vi "LOAD_CONFIG.vi"() -> (3 "출력 클러스터":T1)   [LabVIEW 2019]
uses:
  <vilib>/imath/engines/lvmath/Plug In/Control Design/BuiltInFunctions/tf/NIMS_CD_tf(num,den,Ts).vi
  <vilib>/imath/engines/lvmath2/RunTimeEngine/NodeEndStatement/NIMS_NodeEndStatement_Output.vi
  <vilib>/imath/engines/lvmath2/RunTimeEngine/ErrorHandling/NIMS_Finalize Error.vi
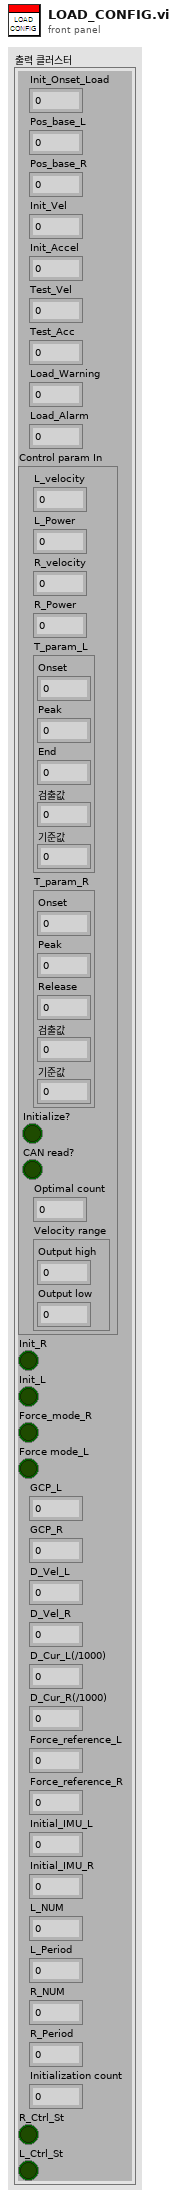
[diagram p1: front panel]
types:
  T1 = cluster{"Init_Onset_Load":sgl, "Pos_base_L":sgl, "Pos_base_R":sgl, "Init_Vel":i32, "Init_Accel":u32, "Test_Vel":i32, "Test_Acc":u32, "Load_Warning":sgl, "Load_Alarm":sgl, "Control param In":cluster{"L_velocity":u32, "L_Power":sgl, "R_velocity":u32, "R_Power":sgl, "T_param_L":cluster{"Onset":sgl, "Peak":sgl, "End":sgl, "검출값":sgl, "기준값":sgl}, "T_param_R":cluster{"Onset":sgl, "Peak":sgl, "Release":sgl, "검출값":sgl, "기준값":sgl}, "Initialize?":bool, "CAN read?":bool, "Optimal count":i32, "Velocity range":cluster{"Output high":dbl, "Output low":dbl}}, "Init_R":bool, "Init_L":bool, "Force_mode_R":bool, "Force mode_L":bool, "GCP_L":sgl, "GCP_R":sgl, "D_Vel_L":sgl, "D_Vel_R":sgl, "D_Cur_L(/1000)":sgl, "D_Cur_R(/1000)":sgl, "Force_reference_L":sgl, "Force_reference_R":sgl, "Initial_IMU_L":sgl, "Initial_IMU_R":sgl, "L_NUM":u32, "L_Period":i16, "R_NUM":u32, "R_Period":i16, "Initialization count":i32, "R_Ctrl_St":bool, "L_Ctrl_St":bool}
  T2 = cluster{"Init_Onset_Load":sgl, "Pos_base_L":sgl, "Pos_base_R":sgl, "Init_Vel":i32, "Init_Accel":u32, "Test_Vel":i32, "Test_Acc":u32, "Load_Warning":sgl, "Load_Alarm":sgl, "Control param In":cluster{"L_velocity":u32, "L_Power":sgl, "R_velocity":u32, "R_Power":sgl, "T_param_L":cluster{"Onset":sgl, "Peak":sgl, "End":sgl, "검출값":sgl, "기준값":sgl}, "T_param_R":cluster{"Onset":sgl, "Peak":sgl, "Release":sgl, "검출값":sgl, "기준값":sgl}, "Initialize?":bool, "CAN read?":bool, "Optimal count":i32, "Velocity range":cluster{"Output high":dbl, "Output low":dbl}}}
  T3 = cluster{"L_velocity":u32, "L_Power":sgl, "R_velocity":u32, "R_Power":sgl, "T_param_L":cluster{"Onset":sgl, "Peak":sgl, "End":sgl, "검출값":sgl, "기준값":sgl}, "T_param_R":cluster{"Onset":sgl, "Peak":sgl, "Release":sgl, "검출값":sgl, "기준값":sgl}, "Initialize?":bool, "CAN read?":bool, "Optimal count":i32, "Velocity range":cluster{"Output high":dbl, "Output low":dbl}}
  T4 = enum16{"open", "replace", "create", "open or create", "replace or create", "replace or create with confirmation"}
  T5 = cluster{"Onset":sgl, "Peak":sgl, "End":sgl, "검출값":sgl, "기준값":sgl}
  T6 = cluster{"Onset":sgl, "Peak":sgl, "Release":sgl, "검출값":sgl, "기준값":sgl}
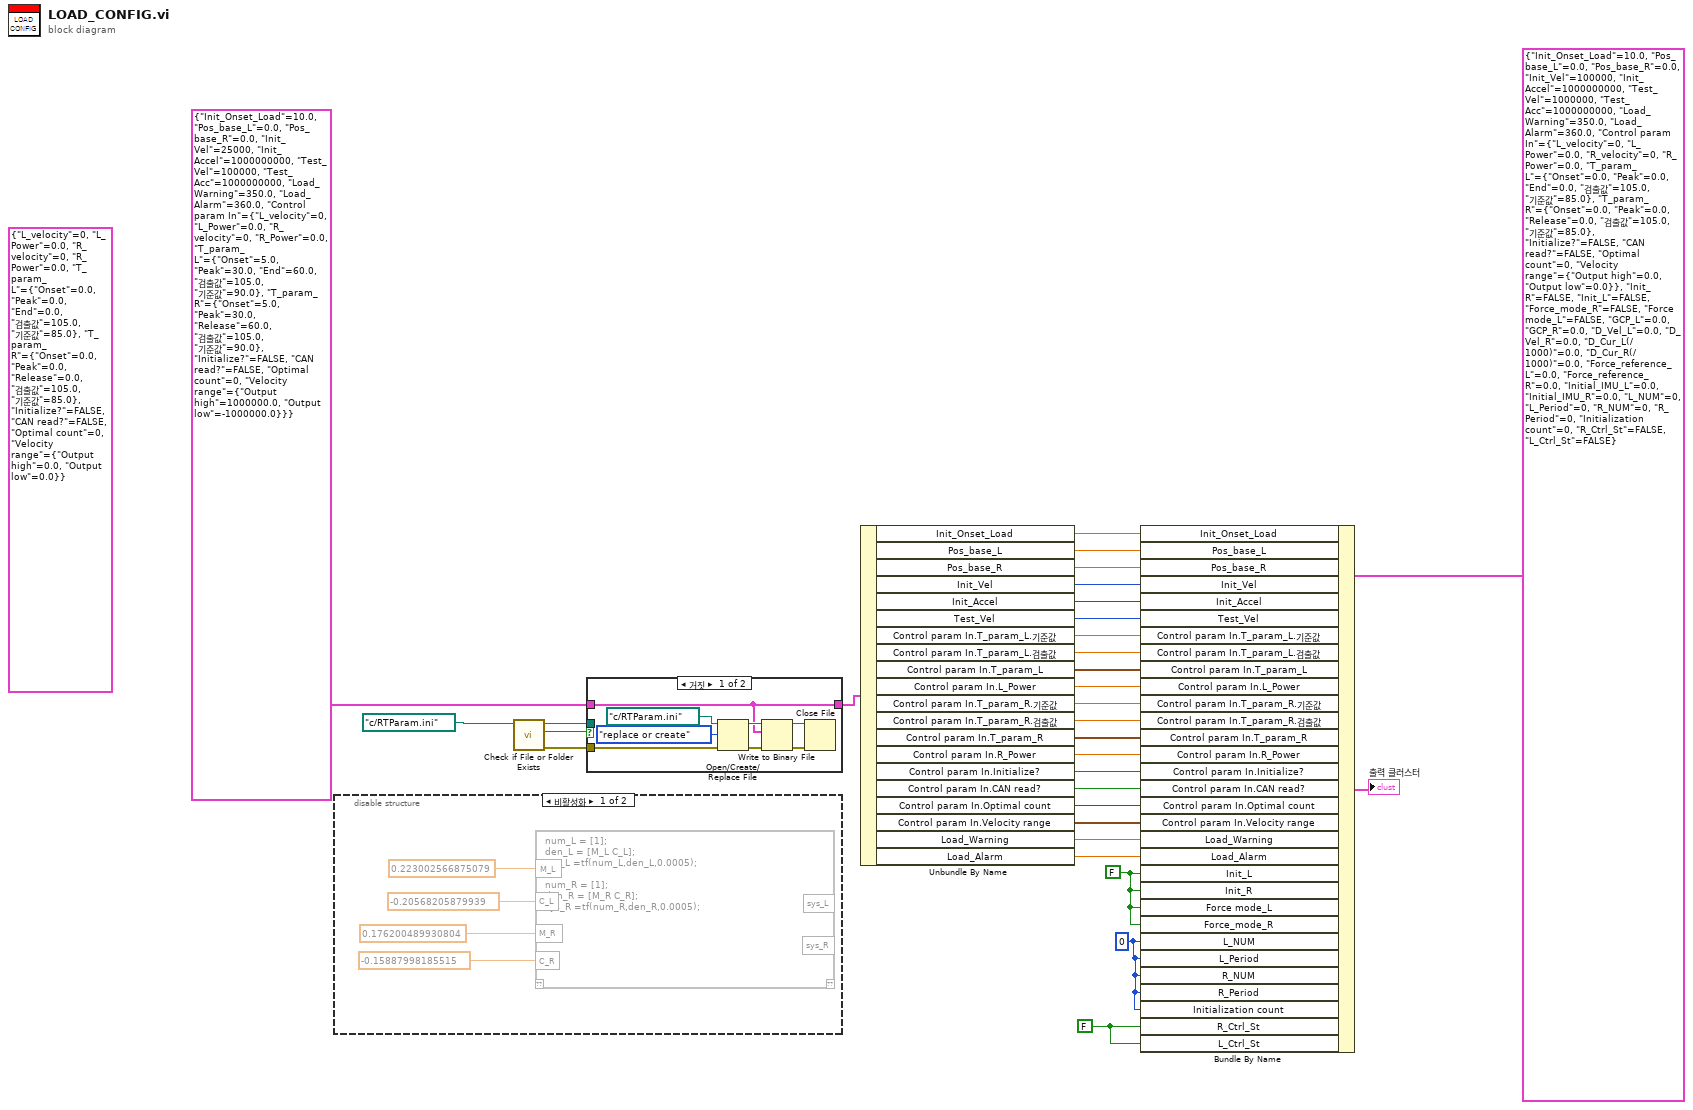
[diagram p0: block diagram]
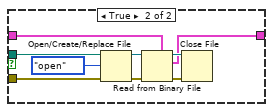
[diagram p3: hidden frame]
diagram:
  w2 = FALSE ("R_Ctrl_St")
  w4 = u32 0 ("L_NUM")
  (unwired) T3 {"L_velocity"=0, "L_Power"=0.0, "R_velocity"=0, "R_Power"=0.0, "T_param_L"={"Onset"=0.0, "Peak"=0.0, "End"=0.0, "검출값"=105.0, "기준값"=85.0}, "T_param_R"={"Onset"=0.0, "Peak"=0.0, "Release"=0.0, "검출값"=105.0, "기준값"=85.0}, "Initialize?"=FALSE, "CAN read?"=FALSE, "Optimal count"=0, "Velocity range"={"Output high"=0.0, "Output low"=0.0}} ("Control param In")
  w3 = FALSE
  n1 = disable-structure shown="비활성화" {
    frame Disabled {
      # "Discrete system transfer function"
      n2 = mathscript code="num_L = [1];\nden_L = [M_L C_L];\nsys_L =tf(num_L,den_L,0.0005);\n\nnum_R = [1];\nden_R = [M_R C_R];\nsys_R =tf(num_R,den_R,0.0005);"("M_L"=0.223002566875079, "C_L"=-0.20568205879939, "M_R"=0.176200489930804 ("M_L"), "C_R"=-0.15887998185515 ("C_L")) -> ()  [unwired: 1 in, 3 out]
    }
    frame Enabled {
    }
  }
  n3 = call <vilib>:"Check if File or Folder Exists.vi"("path"=path "c:/RTParam.ini" ("파일 경로(대화 상자 사용)")) -> ("error out"=w8:errorcluster, "file or folder exists?"=w10:bool, "dup path"=w9:path)  [unwired: 8 in]
  n4 = case shown="거짓" w10 {
    tunnel: T2 {"Init_Onset_Load"=10.0, "Pos_base_L"=0.0, "Pos_base_R"=0.0, "Init_Vel"=25000, "Init_Accel"=1000000000, "Test_Vel"=100000, "Test_Acc"=1000000000, "Load_Warning"=350.0, "Load_Alarm"=360.0, "Control param In"={"L_velocity"=0, "L_Power"=0.0, "R_velocity"=0, "R_Power"=0.0, "T_param_L"={"Onset"=5.0, "Peak"=30.0, "End"=60.0, "검출값"=105.0, "기준값"=90.0}, "T_param_R"={"Onset"=5.0, "Peak"=30.0, "Release"=60.0, "검출값"=105.0, "기준값"=90.0}, "Initialize?"=FALSE, "CAN read?"=FALSE, "Optimal count"=0, "Velocity range"={"Output high"=1000000.0, "Output low"=-1000000.0}}} ("Param_IN") -> [w101 w109]
    tunnel: w9 -> [_ w111]
    tunnel: w8 -> [w102 w110]
    tunnel: [w101 w108] -> w14
    frame False {
      n5 = Open/Create/Replace File(file path (use dialog)=path "c:/RTParam.ini" ("파일 경로(대화 상자 사용)"), error in=w102, operation (0:open)=T4."replace or create" ("동작(0:open)")) -> (refnum out=w107:refnum<file>, error out=w106:errorcluster)  [unwired: 3 in, 1 out]
      n6 = Write to Binary File(file (use dialog)=w107, data=w101, error in=w106) -> (refnum out=w104:refnum<file>, error out=w103:errorcluster)  [unwired: 3 in, 1 out]
      n7 = Close File(refnum=w104, error in=w103) -> ()  [unwired: 2 out]
    }
    frame True {
      n8 = Open/Create/Replace File(file path (use dialog)=w111, error in=w110, operation (0:open)=T4."open" ("동작(0:open)")) -> (refnum out=w116:refnum<file>, error out=w115:errorcluster)  [unwired: 3 in, 1 out]
      n9 = Read from Binary File(5:w109, 8:w115, 11:w116) -> (0:w112:errorcluster, 2:w108:T2, 3:w113:refnum<file>)  [unwired: 3 in, 1 out]
      n10 = Close File(refnum=w113, error in=w112) -> ()  [unwired: 2 out]
    }
  }
  n11 = Unbundle By Name(w14) -> ("Init_Onset_Load"=w31:sgl, "Pos_base_L"=w30:sgl, "Pos_base_R"=w29:sgl, "Init_Vel"=w28:i32, "Init_Accel"=w27:u32, "Test_Vel"=w26:i32, "Control param In.T_param_L.기준값"=w25:sgl, "Control param In.T_param_L.검출값"=w24:sgl, "Control param In.T_param_L"=w23:T5, "Control param In.L_Power"=w22:sgl, "Control param In.T_param_R.기준값"=w21:sgl, "Control param In.T_param_R.검출값"=w20:sgl, "Control param In.T_param_R"=w19:T6, "Control param In.R_Power"=w18:sgl, "Control param In.Initialize?"=w6:bool, "Control param In.CAN read?"=w17:bool, "Control param In.Optimal count"=w16:i32, "Control param In.Velocity range"=w15:cluster{"Output high":dbl, "Output low":dbl}, "Load_Warning"=w13:sgl, "Load_Alarm"=w12:sgl)
  n12 = Bundle By Name(cluster=T1 {"Init_Onset_Load"=10.0, "Pos_base_L"=0.0, "Pos_base_R"=0.0, "Init_Vel"=100000, "Init_Accel"=1000000000, "Test_Vel"=1000000, "Test_Acc"=1000000000, "Load_Warning"=350.0, "Load_Alarm"=360.0, "Control param In"={"L_velocity"=0, "L_Power"=0.0, "R_velocity"=0, "R_Power"=0.0, "T_param_L"={"Onset"=0.0, "Peak"=0.0, "End"=0.0, "검출값"=105.0, "기준값"=85.0}, "T_param_R"={"Onset"=0.0, "Peak"=0.0, "Release"=0.0, "검출값"=105.0, "기준값"=85.0}, "Initialize?"=FALSE, "CAN read?"=FALSE, "Optimal count"=0, "Velocity range"={"Output high"=0.0, "Output low"=0.0}}, "Init_R"=FALSE, "Init_L"=FALSE, "Force_mode_R"=FALSE, "Force mode_L"=FALSE, "GCP_L"=0.0, "GCP_R"=0.0, "D_Vel_L"=0.0, "D_Vel_R"=0.0, "D_Cur_L(/1000)"=0.0, "D_Cur_R(/1000)"=0.0, "Force_reference_L"=0.0, "Force_reference_R"=0.0, "Initial_IMU_L"=0.0, "Initial_IMU_R"=0.0, "L_NUM"=0, "L_Period"=0, "R_NUM"=0, "R_Period"=0, "Initialization count"=0, "R_Ctrl_St"=FALSE, "L_Ctrl_St"=FALSE} ("Param_IN"), "Init_Onset_Load"=w31, "Pos_base_L"=w30, "Pos_base_R"=w29, "Init_Vel"=w28, "Init_Accel"=w27, "Test_Vel"=w26, "Control param In.T_param_L.기준값"=w25, "Control param In.T_param_L.검출값"=w24, "Control param In.T_param_L"=w23, "Control param In.L_Power"=w22, "Control param In.T_param_R.기준값"=w21, "Control param In.T_param_R.검출값"=w20, "Control param In.T_param_R"=w19, "Control param In.R_Power"=w18, "Control param In.Initialize?"=w6, "Control param In.CAN read?"=w17, "Control param In.Optimal count"=w16, "Control param In.Velocity range"=w15, "Load_Warning"=w13, "Load_Alarm"=w12, "Init_L"=w3, "Init_R"=w3, "Force mode_L"=w3, "Force_mode_R"=w3, "L_NUM"=w4, "L_Period"=w4, "R_NUM"=w4, "R_Period"=w4, "Initialization count"=w4, "R_Ctrl_St"=w2, "L_Ctrl_St"=w2) -> (→"출력 클러스터":T1)
